vi "Exclude DQMH default Libraries.vi"(11 "name":string) -> (3 "Is not a DQMH Default Lib?":bool)   [LabVIEW 2020, in "SimpleDependencyInspector.lvlib"]
uses:
  SimpleDependencyInspector.lvlib
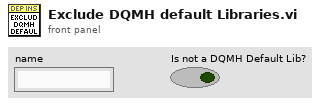
[diagram p1: front panel]
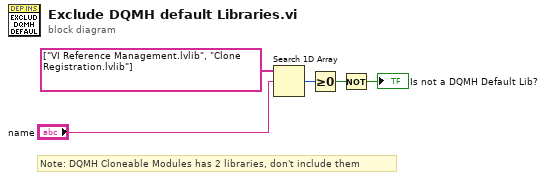
[diagram p0: block diagram]
diagram:
  # "Note: DQMH Cloneable Modules has 2 libraries, don't include them"
  n1 = Search 1D Array(1D array=string[] ["VI Reference Management.lvlib", "Clone Registration.lvlib"], element="name") -> (index of element=w2:i32)  [unwired: 1 in]
  n2 = Greater Or Equal To 0?(x=w2) -> (x >= 0?=w1:bool)
  n3 = Not(x=w1) -> (.not. x?=→"Is not a DQMH Default Lib?":bool)
